vi "Read Sigle Bool.vi"(8 "error in (no error)":errorcluster, 11 "Tags":string) -> (0 "error out":errorcluster, 2 "Boolean":bool, 3 "Siemens Ctr out":T1)   [LabVIEW 2014]
uses:
  Simatic S7.lvlib
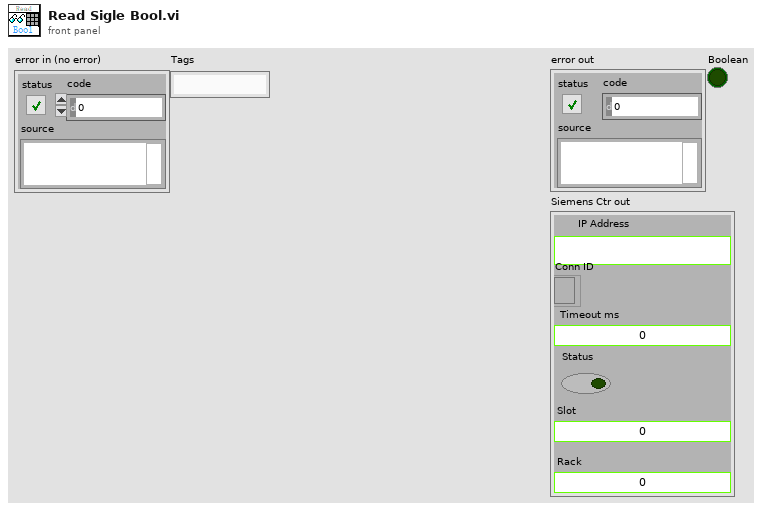
[diagram p1: front panel]
types:
  T1 = typedef "Simatic S7.lvlib/Siemens Ref.ctl" = cluster{"IP Address ":string, "Conn ID":refnum<k5>, "Timeout ms":i32, "Status":bool, "Slot":u16, "Rack":u16}
  T2 = typedef "Simatic S7.lvlib/Operation Siemens Ref.ctl" = enum16{"Init", "Add Ref", "Get Ref", "Set Error", "Close Close"}
  T3 = typedef "PLC Address.ctl" = cluster{"Address Areas":u8, "Data Type":enum8{"Bit", "Byte", "int", "Word", "Dint", "Dword", "Real", "String"}, "DB.No":u16, "Byte":u32, "Length":u16, "Item":u16}
  T4 = typedef "Semaphore RefNum" = refnum<k1>
  T5 = typedef "Simatic S7.lvlib/Op ip address.ctl" = enum16{"Init", "Add IP", "Get IP"}
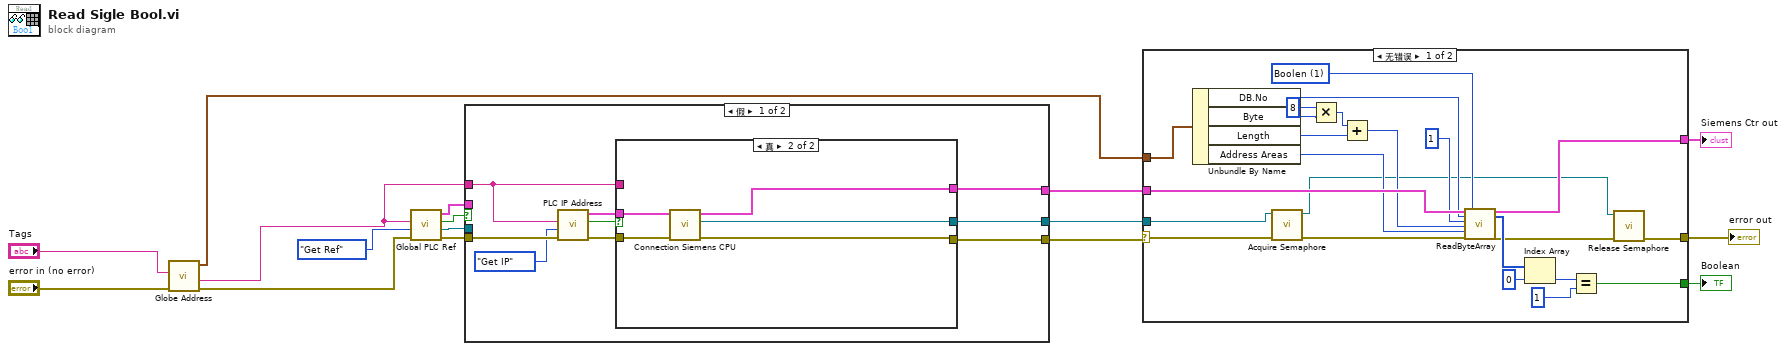
[diagram p0: block diagram]
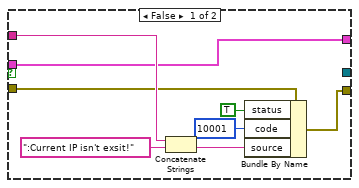
[diagram p3: hidden frame]
diagram:
  n1 = call "Globe Address.vi"("error in (no error)"="error in (no error)", "Tag"="Tags") -> ("error out"=w7:errorcluster, "IP"=w6:string, "ddress"=w4:T3)  [unwired: 6 in, 1 out]
  n2 = call "Global PLC Ref.vi"("error in (no error)"=w7, "Operation Siemens Ref"=Operation_Siemens_Ref."Get Ref", "IP Address"=w6) -> ("error out"=w14:errorcluster, "semaphore"=w12:T4, "Boolean"=w15:bool, "Siemens Ctr out"=w13:T1)  [unwired: 4 in, 1 out]
  n3 = case shown="假" w15 {
    tunnel: w14 -> [w25 w41]
    tunnel: w6 -> [w21 _]
    tunnel: [w19 w41] -> w11
    tunnel: [w18 w39] -> w10
    tunnel: [w17 w40] -> w9
    tunnel: w13 -> [_ w40]
    tunnel: w12 -> [_ w39]
    frame False {
      n4 = call "PLC IP Address.vi"("error in (no error)"=w25, "Operationip"=Op_ip_address."Get IP", "IP Address"=w21) -> ("error out"=w22:errorcluster, "Boolean"=w23:bool, "Siemens Ctr out"=w20:T1)  [unwired: 6 in]
      n5 = case shown="真" w23 {
        tunnel: w22 -> [w31 w38]
        tunnel: w21 -> [w32 _]
        tunnel: w20 -> [w26 w37]
        tunnel: [w27 w36] -> w19
        tunnel: [_ w35] -> w18
        tunnel: [w26 w34] -> w17
        frame False {
          n6 = Concatenate Strings(w32, ":Current IP isn't exsit!") -> (w29:string)
          n7 = Bundle By Name(cluster=w31, "status"=TRUE, "code"=10001, "source"=w29) -> (w27:errorcluster)
        }
        frame True {
          n8 = call "Connection Siemens CPU.vi"("error in (no error)"=w38, "Siemens Ctr in"=w37) -> ("error out"=w36:errorcluster, "semaphore"=w35:T4, "Siemens Ctr out"=w34:T1)  [unwired: 7 in]
        }
      }
    }
    frame True {
    }
  }
  n9 = case shown="无错误" w11 {
    selector: w11 -> [w64 w66]
    tunnel: w10 -> [w57 _]
    tunnel: w9 -> [w62 w65]
    tunnel: w4 -> [w61 _]
    tunnel: [w43 w66] -> w3
    tunnel: [w50 w65] -> w2
    tunnel: [w45 _] -> w1
    frame No Error {
      w60 = u8 1 items=["Boolen"=1, "Byte"=2] ("Bit/Byte")
      n10 = Unbundle By Name(w61) -> ("DB.No"=w59:u16, "Byte"=w56:u32, "Length"=w53:u16, "Address Areas"=w51:u8)
      n11 = call <vilib>:"Acquire Semaphore.vi"("error in (no error)"=w64, "semaphore"=w57) -> ("error out"=w63:errorcluster, "semaphore out"=w42:T4)  [unwired: 3 in, 1 out]
      n12 = Multiply(x=u32 8, y=w56) -> (x*y=w54:u32)
      n13 = Add(x=w54, y=w53) -> (x+y=w52:u32)
      n14 = call "ReadByteArray.vi"("Siemens Ctr"=w62, "# DB No."=w59, "#items"=u16 1, "Item offset [byte]"=w52, "Address Areas"=w51, "error in (no error)"=w63, "Bit/Byte"=w60) -> ("Siemens Ctr out"=w50:T1, "Byte Array"=w49:u8[], "error out"=w44:errorcluster)  [unwired: 10 in]
      n15 = Index Array(array=w49, index=0) -> (element=w47:u8)
      n16 = Equal?(x=w47, y=u8 1) -> (x = y?=w45:bool)
      n17 = call <vilib>:"Release Semaphore.vi"("error in (no error)"=w44, "semaphore"=w42) -> ("error out"=w43:errorcluster)  [unwired: 4 in, 1 out]
    }
    frame Error {
    }
  }
  "error out" <- w3
  "Siemens Ctr out" <- w2
  "Boolean" <- w1
